vi "Load VIs Into Memory.vi"(0 "Project:Open":refnum<vi>, 11 "error in (no error)":errorcluster) -> (15 "error out":errorcluster)   [LabVIEW 2019, in "SolutionBuilder.lvlib"]
uses:
  SolutionBuilder/SolutionBuilder.lvlib
  <vilib>/Utility/EditLVProj/Edit LVProj.lvlib
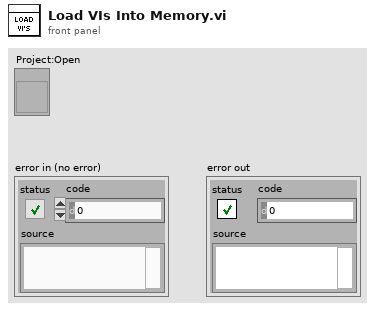
[diagram p1: front panel]
types:
  T1 = enum32{"Invalid", "Standard", "Closed", "Hidden", "Minimized", "Maximized"}
  T2 = typedef "Edit LVProj.lvlib/Library And VI References.ctl" = cluster{"Target Reference":refnum<vi>, "VI References":refnum<vi>[], "Library References":refnum<vi>[]}
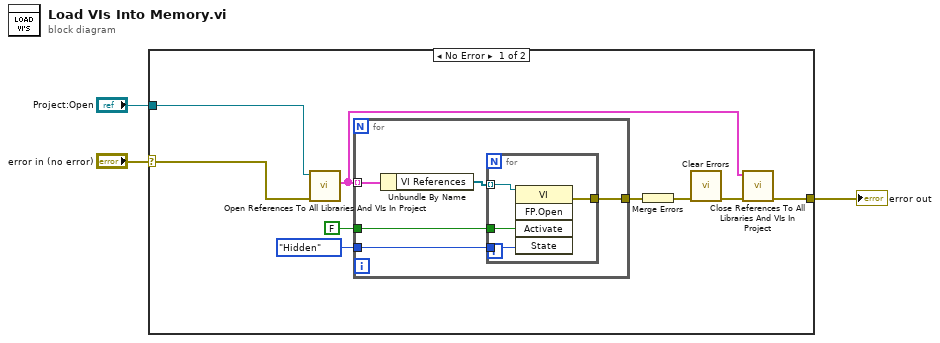
[diagram p0: block diagram]
diagram:
  n1 = case shown="No Error" "error in (no error)" {
    selector: "error in (no error)" -> [w4 w22]
    tunnel: [w6 w22] -> w3
    tunnel: "Project:Open" -> [w5 _]
    frame No Error {
      n2 = call <vilib>:"Open References To All Libraries And VIs In Project.vi"("error in (no error)"=w4, "Project in"=w5) -> ("VI and Library References"=w12:T2[])  [unwired: 7 in, 2 out]
      n3 = for {
        tunnel: w12 -> [w17] mode=indexing
        tunnel: T1."Hidden" ("State") -> [w14]
        tunnel: FALSE ("Activate?") -> [w13]
        tunnel: [w15] -> w11
        n4 = Unbundle By Name(w17) -> ("VI References"=w16:refnum<vi>[])
        n5 = for {
          tunnel: w16 -> [w21] mode=indexing
          tunnel: w14 -> [w19]
          tunnel: w13 -> [w18]
          tunnel: [w20] -> w15
          n6 = invoke class="VI" method="FP.Open"(reference=w21, "Activate"=w18, "State"=w19) -> (error out=w20:errorcluster)  [unwired: 2 in, 4 out]
        }
      }
      n7 = Merge Errors(w11) -> (w8:errorcluster)
      n8 = call <vilib>:"Clear Errors.vi"("error in (no error)"=w8) -> ("error out"=w7:errorcluster)  [unwired: 5 in, 1 out]
      n9 = call <vilib>:"Close References To All Libraries And VIs In Project.vi"("error in (no error)"=w7, "VI and Library References"=w12) -> ("error out"=w6:errorcluster)  [unwired: 9 in]
    }
    frame Error {
    }
  }
  "error out" <- w3
